vi "MainSockets.vi"() -> ()   [LabVIEW 2018]
uses:
  socket REP/socket REP.lvclass
  C:/Users/Denis/Desktop/communication-manager/communication-manager/Socket/Socket.lvclass
  socket REQ/socket REQ.lvclass
  socket SUB/socket SUB.lvclass
  socket PUB/socket PUB.lvclass
  RxTx/CM_RxTx.lvclass
  <vilib>/addons/zeromq/zmq_context.lvclass
  Socket/Socket.lvclass
panel:
  out "error out":errorcluster
  in  "socket PUB.lvclass":refnum<class "socket PUB.lvclass">
  in  "socket SUB.lvclass":refnum<class "socket SUB.lvclass">
  in  "socket REQ.lvclass":refnum<class "socket REQ.lvclass">
  in  "socket REP.lvclass":refnum<class "socket REP.lvclass">
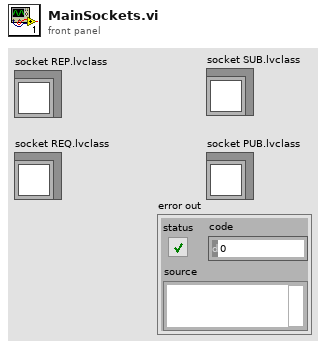
[diagram p1: front panel]
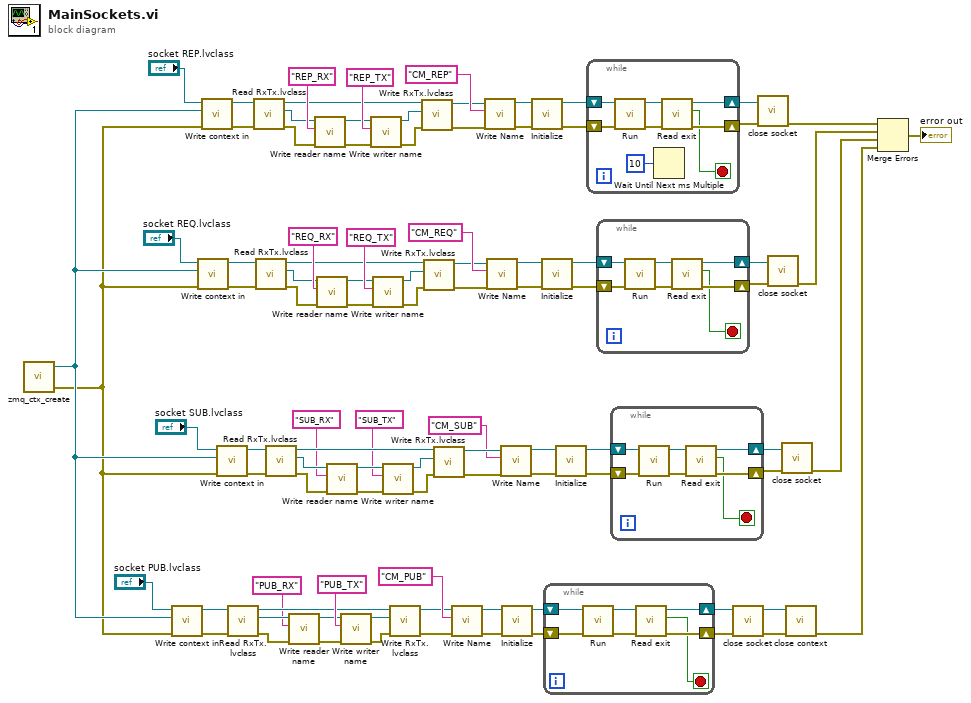
[diagram p0: block diagram]
diagram:
  n1 = call <vilib>:"zmq_ctx_create.vi"() -> ("error out"=w6:errorcluster, "context out"=w7:refnum<class "zmq_context.lvclass">)  [unwired: 4 in]
  n2 = call-dynamic "Write context in.vi"("error in (no error)"=w6, "zeromq.lvlib:ZeroMQ Context"=w7, "Socket in"="socket PUB.lvclass") -> ("error out"=w23:errorcluster, "Socket out"=w22:refnum<class "socket PUB.lvclass">)  [unwired: 7 in]
  n3 = call-dynamic "Write context in.vi"("error in (no error)"=w6, "zeromq.lvlib:ZeroMQ Context"=w7, "Socket in"="socket REQ.lvclass") -> ("error out"=w25:errorcluster, "Socket out"=w24:refnum<class "socket REQ.lvclass">)  [unwired: 7 in]
  n4 = call-dynamic "Write context in.vi"("error in (no error)"=w6, "zeromq.lvlib:ZeroMQ Context"=w7, "Socket in"="socket REP.lvclass") -> ("error out"=w18:errorcluster, "Socket out"=w19:refnum<class "socket REP.lvclass">)  [unwired: 7 in]
  n5 = call-dynamic "Write context in.vi"("error in (no error)"=w6, "zeromq.lvlib:ZeroMQ Context"=w7, "Socket in"="socket SUB.lvclass") -> ("error out"=w20:errorcluster, "Socket out"=w21:refnum<class "socket SUB.lvclass">)  [unwired: 7 in]
  n6 = call-dynamic "Read RxTx.lvclass.vi"("error in (no error)"=w23, "Socket in"=w22) -> ("error out"=w86:errorcluster, "RxTx.lvclass"=w90:refnum<class "CM_RxTx.lvclass">, "Socket out"=w87:refnum<class "socket PUB.lvclass">)  [unwired: 7 in]
  n7 = call-dynamic "Read RxTx.lvclass.vi"("error in (no error)"=w18, "Socket in"=w19) -> ("error out"=w37:errorcluster, "RxTx.lvclass"=w41:refnum<class "CM_RxTx.lvclass">, "Socket out"=w38:refnum<class "socket REP.lvclass">)  [unwired: 7 in]
  n8 = call-dynamic "Read RxTx.lvclass.vi"("error in (no error)"=w25, "Socket in"=w24) -> ("error out"=w53:errorcluster, "RxTx.lvclass"=w57:refnum<class "CM_RxTx.lvclass">, "Socket out"=w54:refnum<class "socket REQ.lvclass">)  [unwired: 7 in]
  n9 = call-dynamic "Read RxTx.lvclass.vi"("error in (no error)"=w20, "Socket in"=w21) -> ("error out"=w68:errorcluster, "RxTx.lvclass"=w64:refnum<class "CM_RxTx.lvclass">, "Socket out"=w67:refnum<class "socket SUB.lvclass">)  [unwired: 7 in]
  n10 = call-dynamic "Write reader name.vi"("error in (no error)"=w86, "RX name"="PUB_RX" ("reader name"), "RxTx in"=w90) -> ("error out"=w85:errorcluster, "RxTx out"=w89:refnum<class "CM_RxTx.lvclass">)  [unwired: 7 in]
  n11 = call-dynamic "Write reader name.vi"("error in (no error)"=w37, "RX name"="REP_RX" ("reader name"), "RxTx in"=w41) -> ("error out"=w36:errorcluster, "RxTx out"=w40:refnum<class "CM_RxTx.lvclass">)  [unwired: 7 in]
  n12 = call-dynamic "Write reader name.vi"("error in (no error)"=w53, "RX name"="REQ_RX" ("reader name"), "RxTx in"=w57) -> ("error out"=w52:errorcluster, "RxTx out"=w56:refnum<class "CM_RxTx.lvclass">)  [unwired: 7 in]
  n13 = call-dynamic "Write reader name.vi"("error in (no error)"=w68, "RX name"="SUB_RX" ("reader name"), "RxTx in"=w64) -> ("error out"=w69:errorcluster, "RxTx out"=w65:refnum<class "CM_RxTx.lvclass">)  [unwired: 7 in]
  n14 = call-dynamic "Write writer name.vi"("error in (no error)"=w85, "Tx name"="PUB_TX" ("writer name"), "RxTx in"=w89) -> ("error out"=w84:errorcluster, "RxTx out"=w88:refnum<class "CM_RxTx.lvclass">)  [unwired: 7 in]
  n15 = call-dynamic "Write writer name.vi"("error in (no error)"=w36, "Tx name"="REP_TX" ("writer name"), "RxTx in"=w40) -> ("error out"=w35:errorcluster, "RxTx out"=w39:refnum<class "CM_RxTx.lvclass">)  [unwired: 7 in]
  n16 = call-dynamic "Write writer name.vi"("error in (no error)"=w52, "Tx name"="REQ_TX" ("writer name"), "RxTx in"=w56) -> ("error out"=w51:errorcluster, "RxTx out"=w55:refnum<class "CM_RxTx.lvclass">)  [unwired: 7 in]
  n17 = call-dynamic "Write writer name.vi"("error in (no error)"=w69, "Tx name"="SUB_TX" ("writer name"), "RxTx in"=w65) -> ("error out"=w70:errorcluster, "RxTx out"=w66:refnum<class "CM_RxTx.lvclass">)  [unwired: 7 in]
  n18 = call-dynamic "Write RxTx.lvclass.vi"("error in (no error)"=w84, "RxTx.lvclass"=w88, "Socket in"=w87) -> ("error out"=w26:errorcluster, "Socket out"=w27:refnum<class "socket PUB.lvclass">)  [unwired: 7 in]
  n19 = call-dynamic "Write RxTx.lvclass.vi"("error in (no error)"=w35, "RxTx.lvclass"=w39, "Socket in"=w38) -> ("error out"=w32:errorcluster, "Socket out"=w33:refnum<class "socket REP.lvclass">)  [unwired: 7 in]
  n20 = call-dynamic "Write RxTx.lvclass.vi"("error in (no error)"=w51, "RxTx.lvclass"=w55, "Socket in"=w54) -> ("error out"=w48:errorcluster, "Socket out"=w49:refnum<class "socket REQ.lvclass">)  [unwired: 7 in]
  n21 = call-dynamic "Write RxTx.lvclass.vi"("error in (no error)"=w70, "RxTx.lvclass"=w66, "Socket in"=w67) -> ("error out"=w73:errorcluster, "Socket out"=w72:refnum<class "socket SUB.lvclass">)  [unwired: 7 in]
  n22 = call-dynamic "Write Name.vi"("error in (no error)"=w26, "Name"="CM_PUB", "Socket in"=w27) -> ("error out"=w82:errorcluster, "Socket out"=w83:refnum<class "socket PUB.lvclass">)  [unwired: 7 in]
  n23 = call-dynamic "Write Name.vi"("error in (no error)"=w32, "Name"="CM_REP", "Socket in"=w33) -> ("error out"=w12:errorcluster, "Socket out"=w13:refnum<class "socket REP.lvclass">)  [unwired: 7 in]
  n24 = call-dynamic "Write Name.vi"("error in (no error)"=w48, "Name"="CM_REQ", "Socket in"=w49) -> ("error out"=w10:errorcluster, "Socket out"=w11:refnum<class "socket REQ.lvclass">)  [unwired: 7 in]
  n25 = call-dynamic "Write Name.vi"("error in (no error)"=w73, "Name"="CM_SUB", "Socket in"=w72) -> ("error out"=w8:errorcluster, "Socket out"=w9:refnum<class "socket SUB.lvclass">)  [unwired: 7 in]
  n26 = call-dynamic "Initialize.vi"("error in (no error)"=w82, "socket PUB in"=w83) -> ("error out"=w79:errorcluster, "socket PUB out"=w81:refnum<class "socket PUB.lvclass">)  [unwired: 8 in]
  n27 = call-dynamic "Initialize.vi"("error in (no error)"=w12, "socket REP in"=w13) -> ("error out"=w29:errorcluster, "socket REP out"=w31:refnum<class "socket REP.lvclass">)  [unwired: 8 in]
  n28 = call-dynamic "Initialize.vi"("error in (no error)"=w10, "socket REQ in"=w11) -> ("error out"=w45:errorcluster, "socket REQ out"=w47:refnum<class "socket REQ.lvclass">)  [unwired: 8 in]
  n29 = while {
    shift-right: [w96] -> w80
    shift-left: w81 -> [w100]
    shift-right: [w95] -> w78
    shift-left: w79 -> [w99]
    stop <- w94 stop-if-true
    n30 = call-dynamic "Run.vi"("error in (no error)"=w99, "socket PUB in"=w100) -> ("error out"=w98:errorcluster, "socket PUB out"=w97:refnum<class "socket PUB.lvclass">)  [unwired: 8 in]
    n31 = call-dynamic "Read exit.vi"("error in (no error)"=w98, "Socket in"=w97) -> ("error out"=w95:errorcluster, "exit"=w94:bool, "Socket out"=w96:refnum<class "socket PUB.lvclass">)  [unwired: 7 in]
  }
  n32 = call-dynamic "Initialize.vi"("error in (no error)"=w8, "socket SUB in"=w9) -> ("error out"=w76:errorcluster, "socket SUB out"=w74:refnum<class "socket SUB.lvclass">)  [unwired: 8 in]
  n33 = while {
    shift-right: [w106] -> w30
    shift-left: w31 -> [w108]
    shift-right: [w103] -> w28
    shift-left: w29 -> [w105]
    stop <- w102 stop-if-true
    n34 = call-dynamic "Run.vi"("error in (no error)"=w105, "socket REP in"=w108) -> ("error out"=w104:errorcluster, "socket REP out"=w107:refnum<class "socket REP.lvclass">)  [unwired: 8 in]
    n35 = Wait Until Next ms Multiple(millisecond multiple=u32 10 ("milliseconds to wait")) -> ()  [unwired: 1 out]
    n36 = call-dynamic "Read exit.vi"("error in (no error)"=w104, "Socket in"=w107) -> ("error out"=w103:errorcluster, "exit"=w102:bool, "Socket out"=w106:refnum<class "socket REP.lvclass">)  [unwired: 7 in]
  }
  n37 = while {
    shift-right: [w113] -> w46
    shift-left: w47 -> [w115]
    shift-right: [w110] -> w44
    shift-left: w45 -> [w112]
    stop <- w109 stop-if-true
    n38 = call-dynamic "Run.vi"("error in (no error)"=w112, "socket REQ in"=w115) -> ("error out"=w111:errorcluster, "socket REQ out"=w114:refnum<class "socket REQ.lvclass">)  [unwired: 8 in]
    n39 = call-dynamic "Read exit.vi"("error in (no error)"=w111, "Socket in"=w114) -> ("error out"=w110:errorcluster, "exit"=w109:bool, "Socket out"=w113:refnum<class "socket REQ.lvclass">)  [unwired: 7 in]
  }
  n40 = while {
    shift-right: [w120] -> w75
    shift-left: w74 -> [w122]
    shift-right: [w117] -> w77
    shift-left: w76 -> [w119]
    stop <- w116 stop-if-true
    n41 = call-dynamic "Run.vi"("error in (no error)"=w119, "socket SUB in"=w122) -> ("error out"=w118:errorcluster, "socket SUB out"=w121:refnum<class "socket SUB.lvclass">)  [unwired: 8 in]
    n42 = call-dynamic "Read exit.vi"("error in (no error)"=w118, "Socket in"=w121) -> ("error out"=w117:errorcluster, "exit"=w116:bool, "Socket out"=w120:refnum<class "socket SUB.lvclass">)  [unwired: 7 in]
  }
  n43 = call "close socket.vi"("error in (no error)"=w78, "Socket in"=w80) -> ("error out"=w93:errorcluster, "Socket out"=w92:refnum<class "socket PUB.lvclass">)  [unwired: 8 in]
  n44 = call "close socket.vi"("error in (no error)"=w28, "Socket in"=w30) -> ("error out"=w5:errorcluster)  [unwired: 8 in, 1 out]
  n45 = call "close socket.vi"("error in (no error)"=w44, "Socket in"=w46) -> ("error out"=w4:errorcluster)  [unwired: 8 in, 1 out]
  n46 = call "close socket.vi"("error in (no error)"=w77, "Socket in"=w75) -> ("error out"=w3:errorcluster)  [unwired: 8 in, 1 out]
  n47 = call-dynamic "close context.vi"("error in (no error)"=w93, "Socket in"=w92) -> ("error out"=w2:errorcluster)  [unwired: 8 in, 1 out]
  n48 = Merge Errors(w5, w4, w3, w2) -> (→"error out":errorcluster)
